vi "Play Warning.vi"(8 "error in (no error)":errorcluster, 11 "task ID":T1 format="%.0x") -> (0 "error out":errorcluster, 3 "task ID 2":T1 format="%.0x")   [LabVIEW 2019]
uses:
  <vilib>/sound2/lvsound2.llb/Sound Output Task ID.ctl
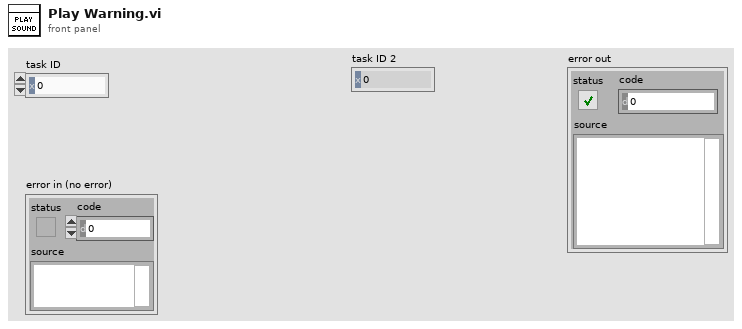
[diagram p1: front panel]
types:
  T1 = typedef "Sound Output Task ID.ctl" = u32
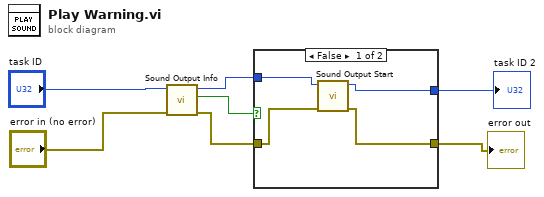
[diagram p0: block diagram]
diagram:
  n1 = call <vilib>:"Sound Output Info.vi"("error in (no error)"="error in (no error)", "task ID"="task ID") -> ("error out"=w2:errorcluster, "is playing?"=w6:bool, "task ID out"=w5:T1)  [unwired: 6 in, 1 out]
  n2 = case shown="False" w6 {
    tunnel: w5 -> [w11 w13]
    tunnel: [w10 w13] -> w4
    tunnel: w2 -> [w9 w12]
    tunnel: [w8 w12] -> w3
    frame False {
      n3 = call <vilib>:"Sound Output Start.vi"("error in (no error)"=w9, "task ID"=w11) -> ("error out"=w8:errorcluster, "task ID out"=w10:T1)  [unwired: 8 in]
    }
    frame True {
    }
  }
  "error out" <- w3
  "task ID 2" <- w4
